vi "Hotkey FGV.vi"(7 "Mode":T2, 8 "error in (no error)":errorcluster, 11 "Hotkey":T1(array[ring])) -> (0 "error out":errorcluster, 2 "Hotkey String out":string, 3 "Hotkey out":T1(array[ring]))   [LabVIEW 2023]
doc: "FGV for setting, starting, and reading a timer."
uses:
  CTLs/FGV Actions.ctl
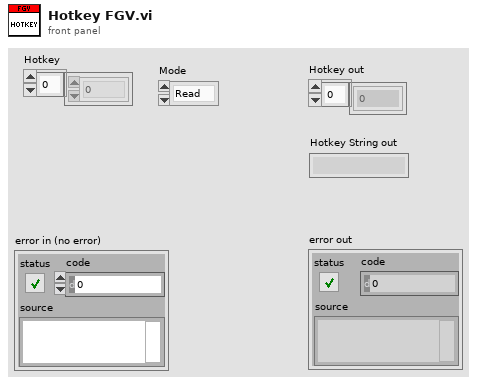
[diagram p1: front panel]
types:
  T1 = enum16{"0", "1", "2", "3", "4", "5", "6", "7", "8", "9", "A", "B", "C", "D", "E", "F", "G", "H", "I", "J", "K", "L", "M", "N", "O", "P", "Q", "R", "S", "T", "U", "V", "W", "X", "Y", "Z", "F1", "F2", "F3", "F4", "F5", "F6", "F7", "F8", "F9", "F10", "F11", "F12", "F13", "F14", "F15", "ADD", "BACK", "BACKSLASH", "CAPITAL", "COMMA", "DECIMAL", "DELETE", "DIVIDE", "DOWN", "END", "EQUALS", "ESCAPE", "GRAVE (`)", "HOME", "INSERT", "LBRACKET", "LCONTROL", "LEFT", "L ALT", "LSHIFT", "LWIN", "MINUS", "MULTIPLY", "NEXT", "NUMLOCK", "NUMPAD_0", "NUMPAD_1", "NUMPAD_2", "NUMPAD_3", "NUMPAD_4", "NUMPAD_5", "NUMPAD_6", "NUMPAD_7", "NUMPAD_8", "NUMPAD_9", "PAUSE", "PERIOD", "PRIOR (PG UP)", "RBRACKET", "RCONTROL", "RETURN", "RIGHT", "R ALT", "RSHIFT", "RWIN", "SCROLL", "SEMICOLON", "SLASH", "SPACE", "SUBTRACT", "TAB", "UP", "ENTER (num pad)", "' (quote)"}[]
  T2 = typedef "FGV Actions.ctl" = enum16{"Read", "Write"}
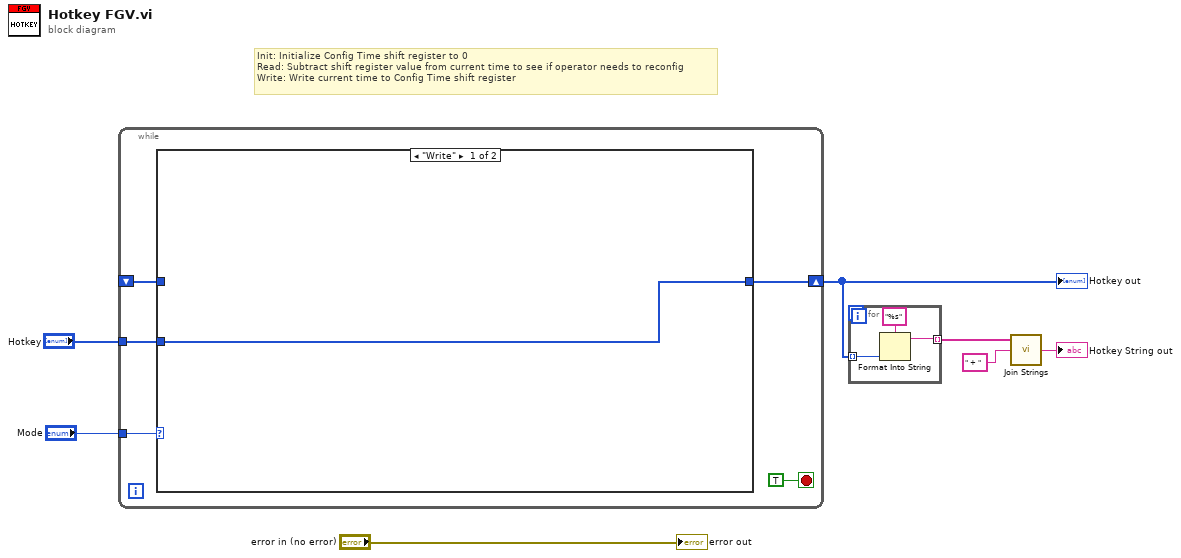
[diagram p0: block diagram]
diagram:
  # "Init: Initialize Config Time shift register to 0\nRead: Subtract shift register value from current time to see if operator needs to reconfig\nWrite: Write current time to Config Time shift register"
  n1 = while {
    tunnel: "Mode" -> [w12]
    shift-right: [w9] -> w2
    shift-left: _ -> [w10]
    tunnel: "Hotkey" -> [w8]
    stop <- TRUE stop-if-true
    n2 = case shown="\"Write\"" w12 {
      tunnel: w10 -> [_ w14]
      tunnel: [w13 w14] -> w9
      tunnel: w8 -> [w13 _]
      frame "Write" {
      }
      frame "Read", Default {
      }
    }
  }
  "Hotkey out" <- w2
  n3 = for {
    tunnel: w2 -> [w16] mode=indexing
    tunnel: [w15] -> w4 mode=indexing
    n4 = Format Into String(format string="%s", w16) -> (resulting string=w15:string)  [unwired: 2 in, 1 out]
  }
  n5 = call <vilib>:"Join Strings.vi"("Separator (,)"=" + ", "Strings In"=w4) -> ("String"=→"Hotkey String out":string)  [unwired: 1 in]
  "error out" <- "error in (no error)"
